vi "Get Selected Measurements.vi"(0 "Tree control in":refnum<vi>, 5 "Measurement file Tags":string[](array[string]), 11 "error in (no error)":errorcluster) -> (4 "Tree control out":refnum<vi>, 6 "Measurement Plug-ins":string[][](array[string]), 15 "error out":errorcluster)   [LabVIEW 2021, in "Migrator.lvlib"]
uses:
  Migrator.lvlib
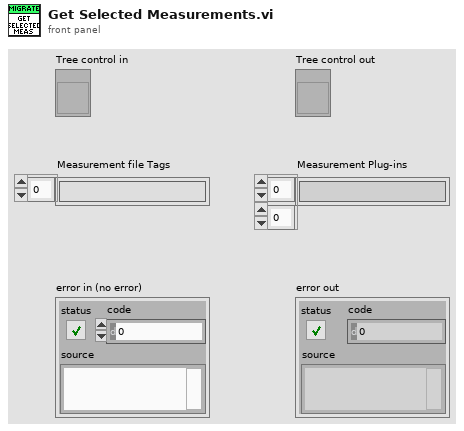
[diagram p1: front panel]
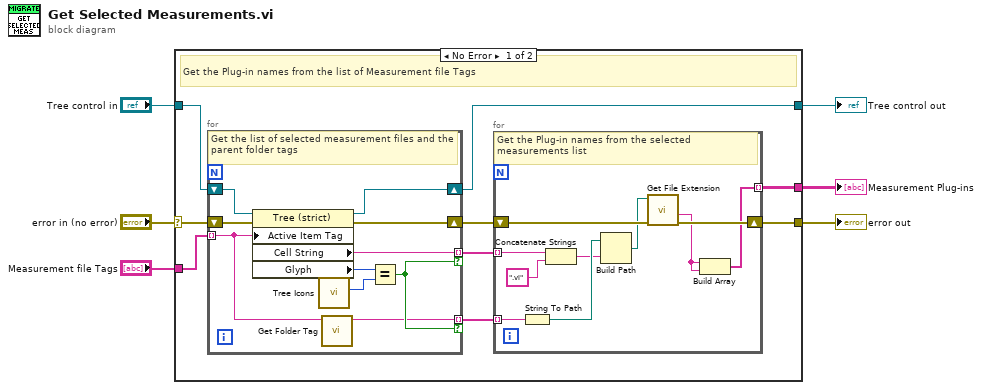
[diagram p0: block diagram]
diagram:
  n1 = case shown="No Error" "error in (no error)" {
    selector: "error in (no error)" -> [w13 w37]
    tunnel: [w8 w37] -> w5
    tunnel: "Tree control in" -> [w15 w36]
    tunnel: "Measurement file Tags" -> [w14 _]
    tunnel: [w10 w36] -> w2
    tunnel: [w7 _] -> w1
    frame No Error {
      # "Get the Plug-in names from the list of Measurement file Tags"
      n2 = for {
        tunnel: w14 -> [w27] mode=indexing
        tunnel: [w26] -> w9 mode=indexing if=w31
        tunnel: [w32] -> w12 mode=indexing if=w31
        shift-right: [w30] -> w11
        shift-left: w13 -> [w29]
        shift-right: [w28] -> w10
        shift-left: w15 -> [w35]
        # "Get the list of selected measurement files and the parent folder tags"
        n3 = property class="Tree (strict)"(reference=w35, error in=w29, "Active Item Tag"=w27) -> (reference out=w28:refnum<vi>, error out=w30:errorcluster, "Cell String"=w32:string, "Glyph"=w33:i32)
        n4 = call "Tree Icons.vi"() -> ("Selected"=w34:i32)  [unwired: 6 in, 1 out]
        n5 = call "Get Folder Tag.vi"("Selected cell Tag"=w27) -> ("Folder Tag"=w26:string)  [unwired: 6 in]
        n6 = Equal?(x=w33, y=w34) -> (x = y?=w31:bool)
      }
      n7 = for {
        tunnel: w12 -> [w24] mode=indexing
        shift-right: [w20] -> w8
        shift-left: w11 -> [w21]
        tunnel: [w18] -> w7 mode=indexing
        tunnel: w9 -> [w17] mode=indexing
        # "Get the Plug-in names from the selected measurements list"
        n8 = String To Path(string=w17) -> (path=w25:path)
        n9 = Concatenate Strings(w24, ".vi" ("string")) -> (w22:string)
        n10 = Build Path(base path=w25, name or relative path=w22) -> (appended path=w19:path)
        n11 = call <vilib>:"Get File Extension.vi"("error in (no error)"=w21, "file"=w19) -> ("error out"=w20:errorcluster, "filename without extension"=w16:string)  [unwired: 5 in, 3 out]
        n12 = Build Array(w16, w16) -> (w18:string[])
      }
    }
    frame Error {
      # "Pass"
    }
  }
  "error out" <- w5
  "Measurement Plug-ins" <- w1
  "Tree control out" <- w2
